vi "Write Trigger Core.vi"(8 "error in (no error)":errorcluster, 10 "PV":refnum<class "PV.lvclass">, 11 "BNT_SLTagConnection in":refnum<class "BNT_SLTagConnection.lvclass">) -> (0 "error out":errorcluster, 3 "BNT_SLTagConnection out":refnum<class "BNT_SLTagConnection.lvclass">)   [LabVIEW 2019, in "BNT_SLTagConnection.lvlib" / "BNT_SLTagConnection.lvclass"]
doc: "Publish a process variable to trigger a paramater less message."
uses:
  BNT_SLTagConnection.lvclass
  CSPP_Core/Classes/CSPP_ProcessVariables/ProcessVariable/PV.lvclass
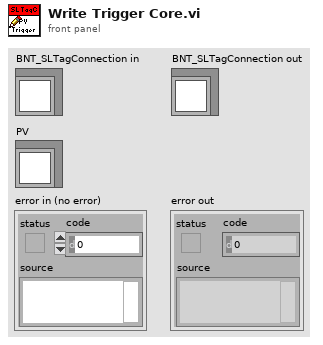
[diagram p1: front panel]
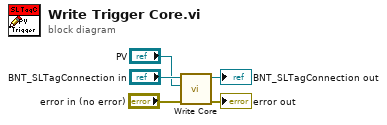
[diagram p0: block diagram]
diagram:
  n1 = call-dynamic "Write Core.vi"("error in"="error in (no error)", "PV"="PV", "BNT_SLTagConnection in"="BNT_SLTagConnection in") -> ("error out"=→"error out":errorcluster, "BNT_SLTagConnection out"=→"BNT_SLTagConnection out":refnum<class "BNT_SLTagConnection.lvclass">)  [unwired: 6 in, 1 out]
